vi "Receiver UI.vi"() -> ()   [LabVIEW 2021, in "Receiver.lvclass"]
uses:
  Receiver.lvclass
  Controls/Operation.ctl
  Controls/State Cluster.ctl
  Controls/User Event Operation.ctl
  Controls/Receiver Data Cluster.ctl
  Downloads/Sample PC Template/Sample PC Template/Typedefs/Data.ctl
  Downloads/Sample PC Template/Sample PC Template/Sample PC Template.lvlib
panel:
  out "Receiver UI Trigered":bool
  out "Data":variant
  out "error out":errorcluster
  in  "error in (no error)":errorcluster
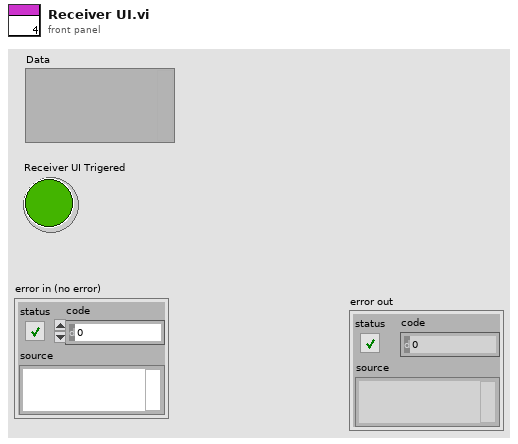
[diagram p1: front panel]
types:
  T1 = typedef "User Event Operation.ctl" = enum16{"Obtain", "Generate", "Release"}
  T2 = typedef "Receiver Data Cluster.ctl" = cluster{"Data":variant, "Receiver UI Triggered":bool}
  T3 = typedef "State Cluster.ctl" = cluster{"State":string, "Data":variant}
  T4 = typedef "Operation.ctl" = enum16{"Create", "Enqueue", "Enqueue N", "Enstack", "Dequeue", "Flush", "Release"}
  T5 = typedef "Sample PC Template.lvlib/Data.ctl" = cluster{"State":string, "Data":variant}
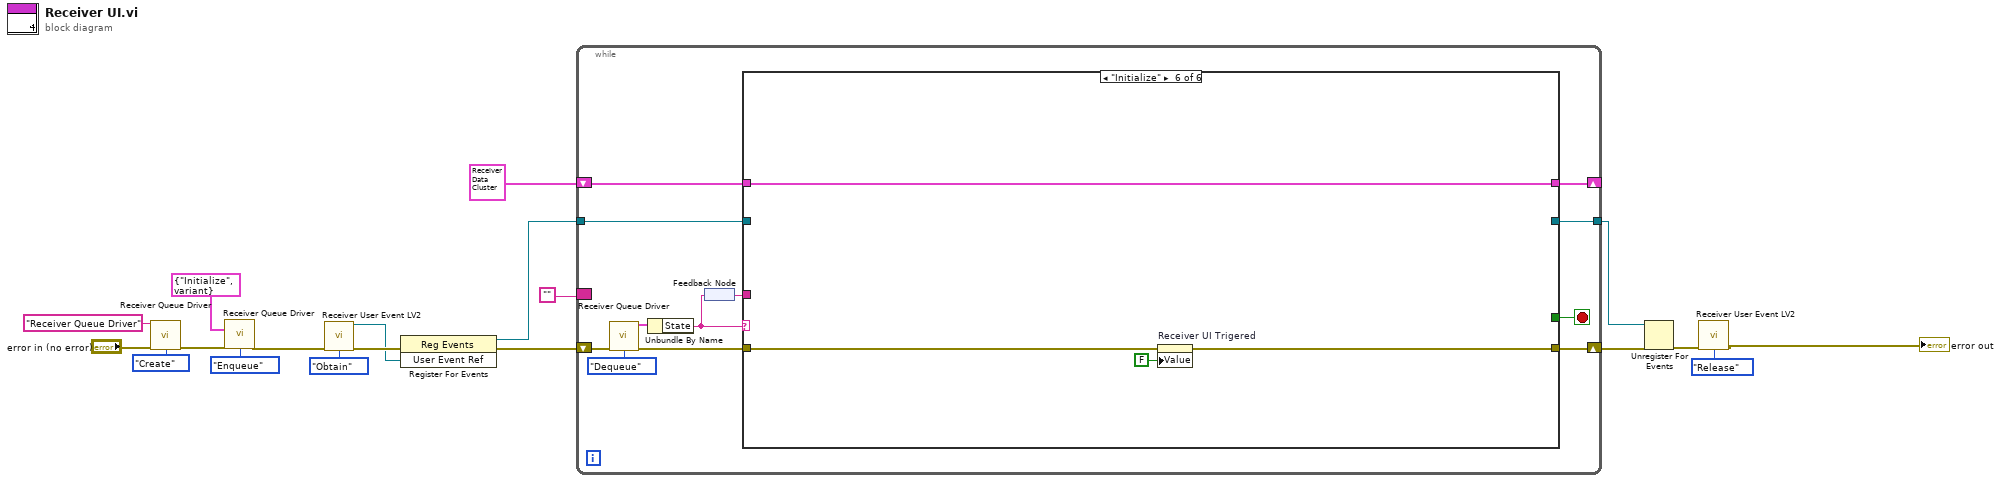
[diagram p0: block diagram]
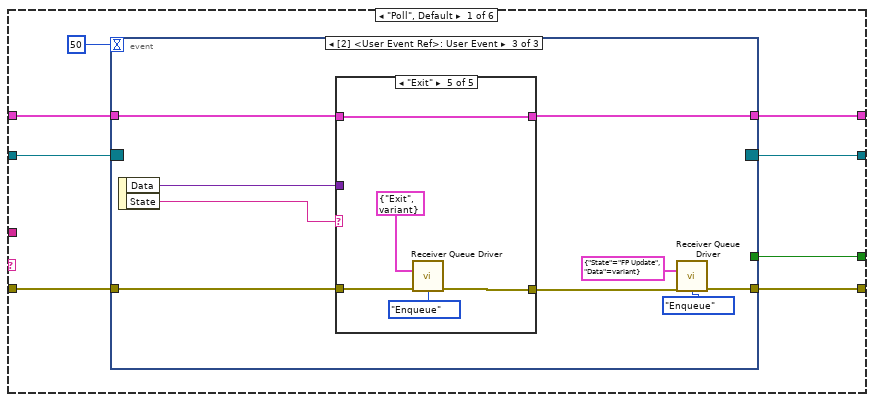
[diagram p2: hidden frame]
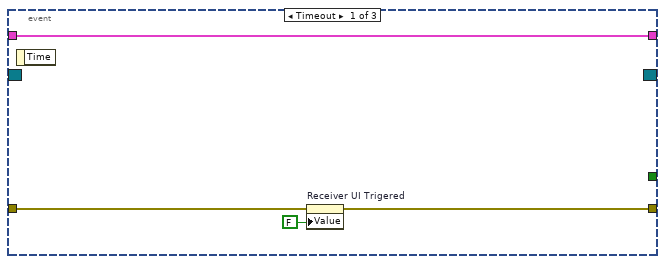
[diagram p3: hidden frame]
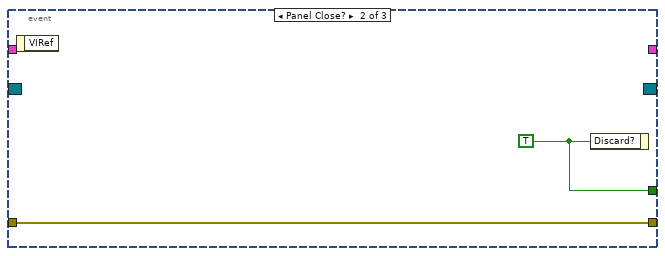
[diagram p4: hidden frame]
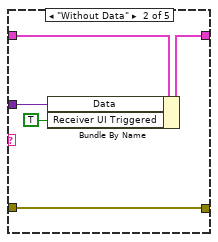
[diagram p6: hidden frame]
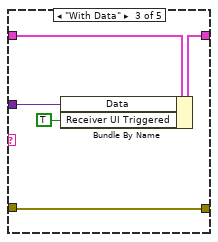
[diagram p7: hidden frame]
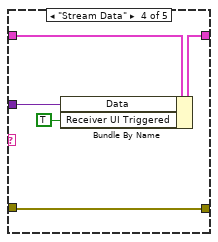
[diagram p8: hidden frame]
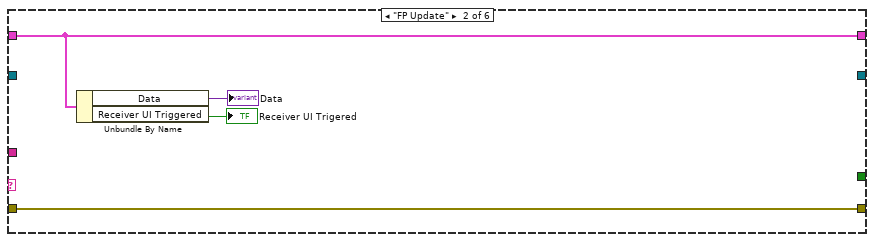
[diagram p9: hidden frame]
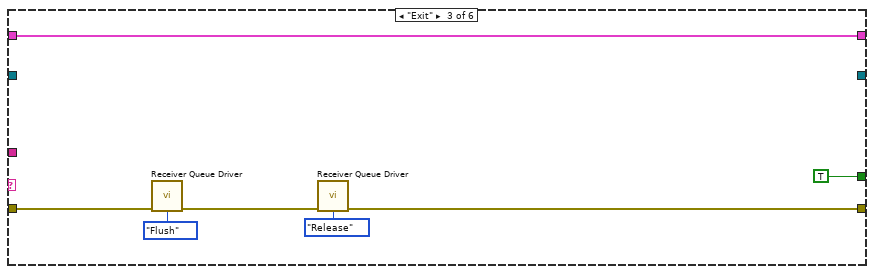
[diagram p10: hidden frame]
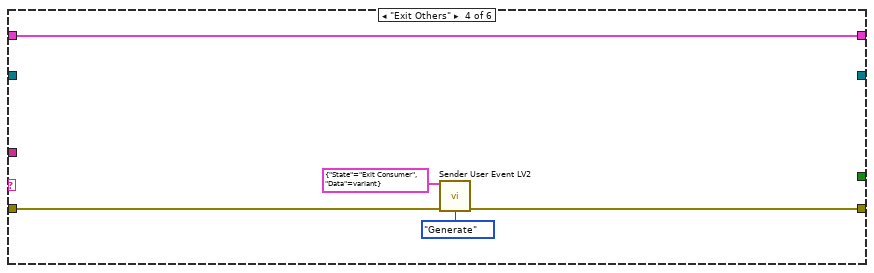
[diagram p11: hidden frame]
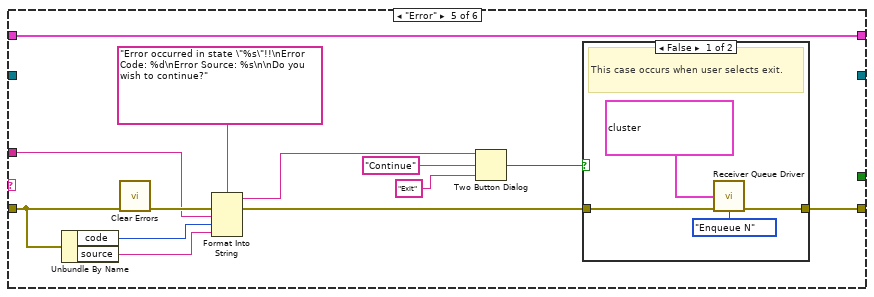
[diagram p12: hidden frame]
diagram:
  n1 = call "Receiver Queue Driver.vi"("Queue Name"="Receiver Queue Driver", "error in (no error)"="error in (no error)", "Operations"=Operation."Create") -> ("error out"=w18:errorcluster)  [unwired: 11 in, 1 out]
  n2 = call "Receiver Queue Driver.vi"("State"=T3 {"State"="Initialize", "Data"=variant}, "error in (no error)"=w18, "Operations"=Operation."Enqueue") -> ("error out"=w12:errorcluster)  [unwired: 11 in, 1 out]
  n3 = call "Receiver User Event LV2.vi"("Error In"=w12, "Operation"=User_Event_Operation."Obtain") -> ("User Event Ref"=w8:refnum<user-event>, "Error Out"=w11:errorcluster)  [unwired: 12 in]
  n4 = register-events(error in=w11, w8) -> (reference out=w7:refnum<event-registration>, error out=w9:errorcluster)  [unwired: 1 in]
  n5 = while {
    border: "" -> [_]
    shift-right: [w25] -> w5
    shift-left: w9 -> [w30]
    tunnel: w7 -> [w23]
    shift-right: [w21] -> _
    shift-left: T2 {"Data"=variant, "Receiver UI Triggered"=FALSE} -> [w22]
    tunnel: [w20] -> w4
    stop <- w24 stop-if-true
    n6 = call "Receiver Queue Driver.vi"("error in (no error)"=w30, "Operations"=Operation."Dequeue") -> ("Dequeued Element"=w29:T3, "error out"=w28:errorcluster)  [unwired: 12 in]
    n7 = Unbundle By Name(w29) -> ("State"=w27:string)
    n8 = feedback-in #1(w27) -> ()
    n9 = feedback #1() -> (w26:string)
    n10 = case shown="\"Initialize\"" w27 {
      tunnel: w28 -> [w39 w80 w87 w92 w97 w113]
      tunnel: w26 -> [_ _ _ _ w94 _]
      tunnel: [w37 w80 w84 w91 w98 w111] -> w25
      tunnel: [w36 _ TRUE ("Discard?") _ _ _] -> w24
      tunnel: w23 -> [w35 _ _ _ _ _]
      tunnel: w22 -> [w34 w78 w81 w88 w93 w114]
      tunnel: [w33 w78 w81 w88 w93 w114] -> w21
      tunnel: [w32 _ _ _ _ _] -> w20
      frame "Poll", Default {
        n11 = event shown="[2] <User Event Ref>: User Event" {
          selector: w35 -> [_ _ _]
          dyn-events: [_ _ _] -> w32
          timeout: 50 -> [_ _ _]
          tunnel: w39 -> [w42 w45 w48]
          tunnel: [w41 w45 w51] -> w37
          tunnel: [_ w44 _] -> w36
          tunnel: w34 -> [w43 _ w54]
          tunnel: [w43 _ w52] -> w33
          event Timeout {
            n12 = event-data() -> ()  [unwired: 1 in, 1 out]
            n13 = property on="Receiver UI Trigered" class="Bool (strict)"(error in=w42, "Value"=FALSE ("Receiver UI Trigered")) -> (error out=w41:errorcluster)  [unwired: 1 in, 1 out]
          }
          event Panel Close? {
            w44 = TRUE ("Discard?")
            n14 = event-data() -> ()  [unwired: 1 in, 1 out]
            n15 = event-data("Discard?"=w44) -> ()  [unwired: 1 in, 1 out]
          }
          event User Event {
            n16 = event-data() -> ("Data"=w53:variant, "State"=w49:string)  [unwired: 1 in]
            n17 = case shown="\"Exit\"" w49 {
              tunnel: w54 -> [w55 w61 w66 w71 w76]
              tunnel: w53 -> [_ w59 w65 w70 _]
              tunnel: [w55 w60 w64 w69 w76] -> w52
              tunnel: w48 -> [w56 w58 w62 w67 w75]
              tunnel: [w56 w58 w62 w67 w74] -> w47
              frame Default {
              }
              frame "Without Data" {
                n18 = Bundle By Name(cluster=w61, "Data"=w59, "Receiver UI Triggered"=TRUE) -> (w60:T2)
              }
              frame "With Data" {
                n19 = Bundle By Name(cluster=w66, "Data"=w65, "Receiver UI Triggered"=TRUE) -> (w64:T2)
              }
              frame "Stream Data" {
                n20 = Bundle By Name(cluster=w71, "Data"=w70, "Receiver UI Triggered"=TRUE) -> (w69:T2)
              }
              frame "Exit" {
                n21 = call "Receiver Queue Driver.vi"("State"=T3 {"State"="Exit", "Data"=variant}, "error in (no error)"=w75, "Operations"=Operation."Enqueue") -> ("error out"=w74:errorcluster)  [unwired: 11 in, 1 out]
              }
            }
            n22 = call "Receiver Queue Driver.vi"("State"=T3 {"State"="FP Update", "Data"=variant}, "error in (no error)"=w47, "Operations"=Operation."Enqueue") -> ("error out"=w51:errorcluster)  [unwired: 11 in, 1 out]
          }
        }
      }
      frame "FP Update" {
        n23 = Unbundle By Name(w78) -> ("Data"=→"Data":variant, "Receiver UI Triggered"=→"Receiver UI Trigered":bool)
      }
      frame "Exit" {
        n24 = call "Receiver Queue Driver.vi"("error in (no error)"=w87, "Operations"=Operation."Flush") -> ("error out"=w85:errorcluster)  [unwired: 12 in, 1 out]
        n25 = call "Receiver Queue Driver.vi"("error in (no error)"=w85, "Operations"=Operation."Release") -> ("error out"=w84:errorcluster)  [unwired: 12 in, 1 out]
      }
      frame "Exit Others" {
        n26 = call "Sender User Event LV2.vi"("Data"=T5 {"State"="Exit Consumer", "Data"=variant}, "Error In"=w92, "Operation"=User_Event_Operation."Generate") -> ("Error Out"=w91:errorcluster)  [unwired: 11 in, 1 out]
      }
      frame "Error" {
        n27 = Unbundle By Name(w97) -> ("code"=w95:i32, "source"=w96:string)
        n28 = call <vilib>:"Clear Errors.vi"("error in (no error)"=w97) -> ("error out"=w105:errorcluster)  [unwired: 5 in, 1 out]
        n29 = Format Into String(format string="Error occurred in state \"%s\"!!\nError Code: %d\nError Source: %s\n\nDo you wish to continue?", error in=w105, w94, w95, w96) -> (resulting string=w103:string, error out=w100:errorcluster)  [unwired: 1 in]
        n30 = Two Button Dialog(message=w103, 1:"Exit" ("F button name (\"Cancel\")"), 2:"Continue" ("T button name (\"OK\")")) -> (T button?=w99:bool)
        n31 = case shown="False" w99 {
          tunnel: w100 -> [w109 w110]
          tunnel: [w108 w110] -> w98
          frame False {
            # "This case occurs when user selects exit."
            n32 = call "Receiver Queue Driver.vi"("State []"=T3[] [{"State"="Exit Others", "Data"=variant}, {"State"="Exit", "Data"=variant}], "error in (no error)"=w109, "Operations"=Operation."Enqueue N") -> ("error out"=w108:errorcluster)  [unwired: 11 in, 1 out]
          }
          frame True {
            # "This case occurs when user selects to continue."
          }
        }
      }
      frame "Initialize" {
        n33 = property on="Receiver UI Trigered" class="Bool (strict)"(error in=w113, "Value"=FALSE ("Receiver UI Trigered")) -> (error out=w111:errorcluster)  [unwired: 1 in, 1 out]
      }
    }
  }
  n34 = Unregister For Events(event registration refnum=w4, error in=w5) -> (error out=w3:errorcluster)
  n35 = call "Receiver User Event LV2.vi"("Error In"=w3, "Operation"=User_Event_Operation."Release") -> ("Error Out"=→"error out":errorcluster)  [unwired: 12 in, 1 out]
